vi "HandleObservationSync.vi"(8 "error in (no error)":errorcluster, 11 "S4GUI in":refnum<class "S4GUI.lvclass">) -> (0 "error out":errorcluster, 3 "S4GUI out":refnum<class "S4GUI.lvclass">)   [LabVIEW 2018, in "S4GUI.lvclass"] (continued)
                }
                frame True {
                  n489 = Concatenate Strings("CHANNEL ERROR " ("string"), ": Not idle. S4GUI:HandleObservationSync.vi state 252." ("Error Msg")) -> (w1188:string)
                }
              }
              n490 = Bundle By Name(cluster=w1171, "Obs_state"=w1169, "Error Msg"=w1162) -> (w1170:refnum<class "S4GUI.lvclass">)
            }
            frame 1 {
              n491 = Build Array(w1198, w1197, w1196, w1195) -> (w1200:bool[])
              n492 = Boolean Array To Number(Boolean array=w1200) -> (number=w1199:u32)
              n493 = Number To Decimal String(number=w1199) -> (decimal integer string=w1193:string)  [unwired: 1 in]
              n494 = Concatenate Strings("CHANNEL ERROR < " ("string"), w1193, ">: Initialization failed. S4GUI:HandleObservationSync.vi state 252." ("Error Msg")) -> (w1192:string)
              n495 = Bundle By Name(cluster=w1203, "Obs_state"=u32 1, "Error Msg"=w1192) -> (w1202:refnum<class "S4GUI.lvclass">)
            }
            frame 2 {
              n496 = Build Array(w1213, w1212, w1211, w1210) -> (w1209:bool[])
              n497 = Boolean Array To Number(Boolean array=w1209) -> (number=w1205:u32)
              n498 = Number To Decimal String(number=w1205) -> (decimal integer string=w1204:string)  [unwired: 1 in]
              n499 = Concatenate Strings("CHANNEL ERROR < " ("string"), w1204, ">:  Invalid Exposition Time. S4GUI:HandleObservationSync.vi state 252." ("Error Msg")) -> (w1207:string)
              n500 = Bundle By Name(cluster=w1216, "Obs_state"=u32 1, "Error Msg"=w1207) -> (w1215:refnum<class "S4GUI.lvclass">)
            }
            frame 3 {
              n501 = Bundle By Name(cluster=w1220, "Obs_state"=u32 1, "Error Msg"="ERROR: Invalid configuration in the channels. S4GUI:HandleObservationSync.vi state 252.") -> (w1219:refnum<class "S4GUI.lvclass">)
            }
          }
        }
        frame 253 {
          # "Sem SyncBox, \ntrigger mode = 0 (internal)\nCom SyncBox\ntrigger mode = 6 (ext. start)"
          n502 = call-dynamic "Read Sync Box.lvclass.vi"("error in (no error)"=w1332, "SPARC4_AC in"=w1331) -> ("error out"=w1334:errorcluster, "Sync Box.lvclass"=w1335:refnum<class "Sync Box.lvclass">, "SPARC4_AC out"=w1330:refnum<class "S4GUI.lvclass">)  [unwired: 7 in]
          n503 = call "Read connection.vi"("error in (no error)"=w1334, "Server in"=w1335) -> ("error out"=w1333:errorcluster, "connection"=w1295:bool)  [unwired: 7 in, 1 out]
          n504 = case shown="True" w1295 {
            tunnel: [u8 6 ("TRIGGER_MODE") u8 0 ("TRIGGER_MODE")] -> w1312
            frame True {
            }
            frame False {
            }
          }
          n505 = call-dynamic "Read AcquisitionA.vi"("error in (no error)"=w1333, "S4ACS_GUI in"=w1330) -> ("error out"=w1317:errorcluster, "Acquisition.lvclass"=w1318:refnum<class "Acquisition.lvclass">, "S4ACS_GUI out"=w1316:refnum<class "S4GUI.lvclass">)  [unwired: 7 in]
          n506 = call-dynamic "Read Channel.vi"("error in (no error)"=w1317, "Acquisition in"=w1318) -> ("error out"=w1300:errorcluster, "Channel.lvclass"=w1299:refnum<class "Channel.lvclass">, "Acquisition out"=w1327:refnum<class "Acquisition.lvclass">)  [unwired: 7 in]
          n507 = call-dynamic "Read Interface.vi"("error in (no error)"=w1300, "Channel in"=w1299) -> ("error out"=w1298:errorcluster, "Interface.lvclass"=w1304:refnum<class "Interface.lvclass">, "Channel out"=w1303:refnum<class "Channel.lvclass">)  [unwired: 7 in]
          n508 = call-dynamic "Get CCD_Config.vi"("error in (no error)"=w1298, "Interface in"=w1304) -> ("error out"=w1311:errorcluster, "output cluster"=w1313:T1, "Interface out"=w1310:refnum<class "Interface.lvclass">)  [unwired: 7 in]
          n509 = Bundle By Name(cluster=w1313, "TRIGGER_MODE"=w1312) -> (w1309:T1)
          n510 = call-dynamic "Set CCD_Config.vi"("error in (no error)"=w1311, "input cluster"=w1309, "Interface in"=w1310) -> ("error out"=w1307:errorcluster, "Interface out"=w1305:refnum<class "Interface.lvclass">)  [unwired: 7 in]
          n511 = Flatten To String(anything=w1309, error in (no error)=w1307) -> (data string=w1308:string, error out=w1306:errorcluster)  [unwired: 2 in, 1 out]
          n512 = call "Write flatted cluster.vi"("error in (no error)"=w1306, "flatted cluster"=w1308, "Interface in"=w1305) -> ("error out"=w1301:errorcluster, "Interface out"=w1302:refnum<class "Interface.lvclass">)  [unwired: 7 in]
          n513 = Increment(x=w1338) -> (x+1=w1337:u32)
          n514 = call-dynamic "Write Interface.vi"("error in (no error)"=w1301, "Interface.lvclass"=w1302, "Channel in"=w1303) -> ("error out"=w1297:errorcluster, "Channel out"=w1296:refnum<class "Channel.lvclass">)  [unwired: 7 in]
          n515 = call-dynamic "Read State Machine.vi"("error in (no error)"=w1297, "Device in"=w1296) -> ("error out"=w1324:errorcluster, "State Machine.lvclass"=w1326:refnum<class "State Machine.lvclass">, "Device out"=w1322:refnum<class "Channel.lvclass">)  [unwired: 7 in]
          n516 = call "Next State.vi"("error in (no error)"=w1324, "New_State"=60, "State Machine in"=w1326) -> ("error out"=w1319:errorcluster, "State Machine out"=w1320:refnum<class "State Machine.lvclass">)  [unwired: 7 in]
          n517 = call-dynamic "Write State Machine.vi"("error in (no error)"=w1319, "State Machine.lvclass"=w1320, "Device in"=w1322) -> ("error out"=w1321:errorcluster, "Device out"=w1323:refnum<class "Channel.lvclass">)  [unwired: 7 in]
          n518 = call-dynamic "Write Channel.vi"("error in (no error)"=w1321, "Channel.lvclass"=w1323, "Acquisition in"=w1327) -> ("error out"=w1314:errorcluster, "Acquisition out"=w1315:refnum<class "Acquisition.lvclass">)  [unwired: 7 in]
          n519 = call-dynamic "Write AcquisitionA.vi"("error in (no error)"=w1314, "Acquisition.lvclass"=w1315, "S4ACS_GUI in"=w1316) -> ("error out"=w1329:errorcluster, "S4ACS_GUI out"=w1328:refnum<class "S4GUI.lvclass">)  [unwired: 7 in]
          n520 = Bundle By Name(cluster=w1328, "Obs_state"=w1337) -> (w1336:refnum<class "S4GUI.lvclass">)
        }
        frame 254 {
          # "Espera terminar a execução do comando atual \nantes de ir ao proximo passo da Observação."
          n521 = call-dynamic "Read AcquisitionA.vi"("error in (no error)"=w1358, "S4ACS_GUI in"=w1359) -> ("error out"=w1364:errorcluster, "Acquisition.lvclass"=w1365:refnum<class "Acquisition.lvclass">, "S4ACS_GUI out"=w1361:refnum<class "S4GUI.lvclass">)  [unwired: 7 in]
          n522 = call-dynamic "Read Channel.vi"("error in (no error)"=w1364, "Acquisition in"=w1365) -> ("error out"=w1356:errorcluster, "Channel.lvclass"=w1355:refnum<class "Channel.lvclass">, "Acquisition out"=w1363:refnum<class "Acquisition.lvclass">)  [unwired: 7 in]
          n523 = call-dynamic "Read State Machine.vi"("error in (no error)"=w1356, "Device in"=w1355) -> ("error out"=w1347:errorcluster, "State Machine.lvclass"=w1349:refnum<class "State Machine.lvclass">, "Device out"=w1353:refnum<class "Channel.lvclass">)  [unwired: 7 in]
          n524 = call-dynamic "Read State.vi"("error in (no error)"=w1347, "State Machine in"=w1349) -> ("error out"=w1346:errorcluster, "State"=w1343:i32, "State Machine out"=w1348:refnum<class "State Machine.lvclass">)  [unwired: 7 in]
          n525 = Equal To 0?(x=w1343) -> (x = 0?=w1345:bool)
          n526 = call-dynamic "Write State Machine.vi"("error in (no error)"=w1346, "State Machine.lvclass"=w1348, "Device in"=w1353) -> ("error out"=w1352:errorcluster, "Device out"=w1354:refnum<class "Channel.lvclass">)  [unwired: 7 in]
          n527 = call-dynamic "Write Channel.vi"("error in (no error)"=w1352, "Channel.lvclass"=w1354, "Acquisition in"=w1363) -> ("error out"=w1360:errorcluster, "Acquisition out"=w1362:refnum<class "Acquisition.lvclass">)  [unwired: 7 in]
          n528 = disable-structure shown="Enabled" {
            disable-tunnel: [u32 299 ("t") w1367] -> w1342
            disable-tunnel: w1341 -> [_ w1368]
            frame Disabled {
            }
            frame Enabled {
              n529 = Increment(x=w1368) -> (x+1=w1367:u32)
            }
          }
          n530 = Select(t=w1342, s=w1345, f=w1341) -> (s? t:f=w1344:u32)
          n531 = call-dynamic "Write AcquisitionA.vi"("error in (no error)"=w1360, "Acquisition.lvclass"=w1362, "S4ACS_GUI in"=w1361) -> ("error out"=w1357:errorcluster, "S4ACS_GUI out"=w1351:refnum<class "S4GUI.lvclass">)  [unwired: 7 in]
          n532 = Bundle By Name(cluster=w1351, "Obs_state"=w1344) -> (w1350:refnum<class "S4GUI.lvclass">)
        }
        frame 255 {
          n533 = call "Read AcquisitionB.vi"("error in (no error)"=w1379, "S4ACS_GUI in"=w1380) -> ("error out"=w1372:errorcluster, "Acquisition.lvclass"=w1373:refnum<class "Acquisition.lvclass">, "S4ACS_GUI out"=w1382:refnum<class "S4GUI.lvclass">)  [unwired: 7 in]
          n534 = call "Read connection.vi"("error in (no error)"=w1372, "Server in"=w1373) -> ("error out"=w1371:errorcluster, "connection"=w1369:bool, "Server out"=w1370:refnum<class "Acquisition.lvclass">)  [unwired: 7 in]
          n535 = case shown="False" w1369 {
            tunnel: w1370 -> [w1390 w1410]
            tunnel: w1371 -> [w1389 w1409]
            tunnel: [w1390 w1407] -> w1383
            tunnel: [w1389 w1406] -> w1381
            tunnel: w1376 -> [w1388 w1399]
            tunnel: [w1384 w1398] -> w1375
            frame False {
              n536 = Increment(x=w1388) -> (x+1=w1387:u32)
              n537 = Increment(x=w1387) -> (x+1=w1386:u32)
              n538 = Increment(x=w1386) -> (x+1=w1385:u32)
              n539 = Increment(x=w1385) -> (x+1=w1384:u32)
            }
            frame True {
              # "configura o canal,\nmas não dispara\na exposicao."
              n540 = call-dynamic "Read Channel.vi"("error in (no error)"=w1409, "Acquisition in"=w1410) -> ("error out"=w1395:errorcluster, "Channel.lvclass"=w1397:refnum<class "Channel.lvclass">, "Acquisition out"=w1408:refnum<class "Acquisition.lvclass">)  [unwired: 7 in]
              n541 = call-dynamic "Write expose.vi"("error in (no error)"=w1395, "expose"=FALSE, "Channel in"=w1397) -> ("error out"=w1394:errorcluster, "Channel out"=w1396:refnum<class "Channel.lvclass">)  [unwired: 7 in]
              n542 = call-dynamic "Read State Machine.vi"("error in (no error)"=w1394, "Device in"=w1396) -> ("error out"=w1403:errorcluster, "State Machine.lvclass"=w1405:refnum<class "State Machine.lvclass">, "Device out"=w1401:refnum<class "Channel.lvclass">)  [unwired: 7 in]
              n543 = call "Next State.vi"("error in (no error)"=w1403, "New_State"=1, "State Machine in"=w1405) -> ("error out"=w1391:errorcluster, "State Machine out"=w1392:refnum<class "State Machine.lvclass">)  [unwired: 7 in]
              n544 = Increment(x=w1399) -> (x+1=w1398:u32)
              n545 = call-dynamic "Write State Machine.vi"("error in (no error)"=w1391, "State Machine.lvclass"=w1392, "Device in"=w1401) -> ("error out"=w1400:errorcluster, "Device out"=w1402:refnum<class "Channel.lvclass">)  [unwired: 7 in]
              n546 = call-dynamic "Write Channel.vi"("error in (no error)"=w1400, "Channel.lvclass"=w1402, "Acquisition in"=w1408) -> ("error out"=w1406:errorcluster, "Acquisition out"=w1407:refnum<class "Acquisition.lvclass">)  [unwired: 7 in]
            }
          }
          n547 = call "Write AcquisitionB.vi"("error in (no error)"=w1381, "Acquisition.lvclass"=w1383, "S4ACS_GUI in"=w1382) -> ("error out"=w1378:errorcluster, "S4ACS_GUI out"=w1377:refnum<class "S4GUI.lvclass">)  [unwired: 7 in]
          n548 = Bundle By Name(cluster=w1377, "Obs_state"=w1375) -> (w1374:refnum<class "S4GUI.lvclass">)
        }
        frame 256 {
          # "Espera terminar a execução do comando atual \nantes de ir ao proximo passo da Observação."
          n549 = call "Read AcquisitionB.vi"("error in (no error)"=w1428, "S4ACS_GUI in"=w1429) -> ("error out"=w1434:errorcluster, "Acquisition.lvclass"=w1435:refnum<class "Acquisition.lvclass">, "S4ACS_GUI out"=w1431:refnum<class "S4GUI.lvclass">)  [unwired: 7 in]
          n550 = call-dynamic "Read Channel.vi"("error in (no error)"=w1434, "Acquisition in"=w1435) -> ("error out"=w1426:errorcluster, "Channel.lvclass"=w1425:refnum<class "Channel.lvclass">, "Acquisition out"=w1433:refnum<class "Acquisition.lvclass">)  [unwired: 7 in]
          n551 = call-dynamic "Read State Machine.vi"("error in (no error)"=w1426, "Device in"=w1425) -> ("error out"=w1417:errorcluster, "State Machine.lvclass"=w1419:refnum<class "State Machine.lvclass">, "Device out"=w1423:refnum<class "Channel.lvclass">)  [unwired: 7 in]
          n552 = call-dynamic "Read State.vi"("error in (no error)"=w1417, "State Machine in"=w1419) -> ("error out"=w1416:errorcluster, "State"=w1413:i32, "State Machine out"=w1418:refnum<class "State Machine.lvclass">)  [unwired: 7 in]
          n553 = call-dynamic "Write State Machine.vi"("error in (no error)"=w1416, "State Machine.lvclass"=w1418, "Device in"=w1423) -> ("error out"=w1422:errorcluster, "Device out"=w1424:refnum<class "Channel.lvclass">)  [unwired: 7 in]
          n554 = call-dynamic "Write Channel.vi"("error in (no error)"=w1422, "Channel.lvclass"=w1424, "Acquisition in"=w1433) -> ("error out"=w1430:errorcluster, "Acquisition out"=w1432:refnum<class "Acquisition.lvclass">)  [unwired: 7 in]
          n555 = Equal To 0?(x=w1413) -> (x = 0?=w1415:bool)
          n556 = disable-structure shown="Enabled" {
            disable-tunnel: [u32 299 ("t") w1437] -> w1411
            disable-tunnel: w1412 -> [_ w1440]
            frame Disabled {
            }
            frame Enabled {
              n557 = Increment(x=w1440) -> (x+1=w1439:u32)
              n558 = Increment(x=w1439) -> (x+1=w1438:u32)
              n559 = Increment(x=w1438) -> (x+1=w1437:u32)
            }
          }
          n560 = Select(t=w1411, s=w1415, f=w1412) -> (s? t:f=w1414:u32)
          n561 = call "Write AcquisitionB.vi"("error in (no error)"=w1430, "Acquisition.lvclass"=w1432, "S4ACS_GUI in"=w1431) -> ("error out"=w1427:errorcluster, "S4ACS_GUI out"=w1421:refnum<class "S4GUI.lvclass">)  [unwired: 7 in]
          n562 = Bundle By Name(cluster=w1421, "Obs_state"=w1414) -> (w1420:refnum<class "S4GUI.lvclass">)
        }
        frame 257 {
          # "Sem SyncBox, \ntrigger mode = 0 (internal)\nCom SyncBox\ntrigger mode = 6 (ext. start)"
          n563 = call-dynamic "Read Sync Box.lvclass.vi"("error in (no error)"=w1478, "SPARC4_AC in"=w1477) -> ("error out"=w1480:errorcluster, "Sync Box.lvclass"=w1481:refnum<class "Sync Box.lvclass">, "SPARC4_AC out"=w1476:refnum<class "S4GUI.lvclass">)  [unwired: 7 in]
          n564 = call "Read connection.vi"("error in (no error)"=w1480, "Server in"=w1481) -> ("error out"=w1479:errorcluster, "connection"=w1442:bool)  [unwired: 7 in, 1 out]
          n565 = case shown="False" w1442 {
            tunnel: [u8 6 ("TRIGGER_MODE") u8 0 ("TRIGGER_MODE")] -> w1441
            frame True {
            }
            frame False {
            }
          }
          n566 = call "Read AcquisitionB.vi"("error in (no error)"=w1479, "S4ACS_GUI in"=w1476) -> ("error out"=w1463:errorcluster, "Acquisition.lvclass"=w1464:refnum<class "Acquisition.lvclass">, "S4ACS_GUI out"=w1462:refnum<class "S4GUI.lvclass">)  [unwired: 7 in]
          n567 = call-dynamic "Read Channel.vi"("error in (no error)"=w1463, "Acquisition in"=w1464) -> ("error out"=w1447:errorcluster, "Channel.lvclass"=w1446:refnum<class "Channel.lvclass">, "Acquisition out"=w1473:refnum<class "Acquisition.lvclass">)  [unwired: 7 in]
          n568 = call-dynamic "Read Interface.vi"("error in (no error)"=w1447, "Channel in"=w1446) -> ("error out"=w1445:errorcluster, "Interface.lvclass"=w1451:refnum<class "Interface.lvclass">, "Channel out"=w1450:refnum<class "Channel.lvclass">)  [unwired: 7 in]
          n569 = call-dynamic "Get CCD_Config.vi"("error in (no error)"=w1445, "Interface in"=w1451) -> ("error out"=w1458:errorcluster, "output cluster"=w1459:T1, "Interface out"=w1457:refnum<class "Interface.lvclass">)  [unwired: 7 in]
          n570 = Bundle By Name(cluster=w1459, "TRIGGER_MODE"=w1441) -> (w1456:T1)
          n571 = call-dynamic "Set CCD_Config.vi"("error in (no error)"=w1458, "input cluster"=w1456, "Interface in"=w1457) -> ("error out"=w1454:errorcluster, "Interface out"=w1452:refnum<class "Interface.lvclass">)  [unwired: 7 in]
          n572 = Flatten To String(anything=w1456, error in (no error)=w1454) -> (data string=w1455:string, error out=w1453:errorcluster)  [unwired: 2 in, 1 out]
          n573 = call "Write flatted cluster.vi"("error in (no error)"=w1453, "flatted cluster"=w1455, "Interface in"=w1452) -> ("error out"=w1448:errorcluster, "Interface out"=w1449:refnum<class "Interface.lvclass">)  [unwired: 7 in]
          n574 = Increment(x=w1484) -> (x+1=w1483:u32)
          n575 = call-dynamic "Write Interface.vi"("error in (no error)"=w1448, "Interface.lvclass"=w1449, "Channel in"=w1450) -> ("error out"=w1444:errorcluster, "Channel out"=w1443:refnum<class "Channel.lvclass">)  [unwired: 7 in]
          n576 = call-dynamic "Read State Machine.vi"("error in (no error)"=w1444, "Device in"=w1443) -> ("error out"=w1470:errorcluster, "State Machine.lvclass"=w1472:refnum<class "State Machine.lvclass">, "Device out"=w1468:refnum<class "Channel.lvclass">)  [unwired: 7 in]
          n577 = call "Next State.vi"("error in (no error)"=w1470, "New_State"=60, "State Machine in"=w1472) -> ("error out"=w1465:errorcluster, "State Machine out"=w1466:refnum<class "State Machine.lvclass">)  [unwired: 7 in]
          n578 = call-dynamic "Write State Machine.vi"("error in (no error)"=w1465, "State Machine.lvclass"=w1466, "Device in"=w1468) -> ("error out"=w1467:errorcluster, "Device out"=w1469:refnum<class "Channel.lvclass">)  [unwired: 7 in]
          n579 = call-dynamic "Write Channel.vi"("error in (no error)"=w1467, "Channel.lvclass"=w1469, "Acquisition in"=w1473) -> ("error out"=w1460:errorcluster, "Acquisition out"=w1461:refnum<class "Acquisition.lvclass">)  [unwired: 7 in]
          n580 = call "Write AcquisitionB.vi"("error in (no error)"=w1460, "Acquisition.lvclass"=w1461, "S4ACS_GUI in"=w1462) -> ("error out"=w1475:errorcluster, "S4ACS_GUI out"=w1474:refnum<class "S4GUI.lvclass">)  [unwired: 7 in]
          n581 = Bundle By Name(cluster=w1474, "Obs_state"=w1483) -> (w1482:refnum<class "S4GUI.lvclass">)
        }
        frame 258 {
          # "Espera terminar a execução do comando atual \nantes de ir ao proximo passo da Observação."
          n582 = call "Read AcquisitionB.vi"("error in (no error)"=w1504, "S4ACS_GUI in"=w1505) -> ("error out"=w1510:errorcluster, "Acquisition.lvclass"=w1511:refnum<class "Acquisition.lvclass">, "S4ACS_GUI out"=w1507:refnum<class "S4GUI.lvclass">)  [unwired: 7 in]
          n583 = call-dynamic "Read Channel.vi"("error in (no error)"=w1510, "Acquisition in"=w1511) -> ("error out"=w1502:errorcluster, "Channel.lvclass"=w1501:refnum<class "Channel.lvclass">, "Acquisition out"=w1509:refnum<class "Acquisition.lvclass">)  [unwired: 7 in]
          n584 = call-dynamic "Read State Machine.vi"("error in (no error)"=w1502, "Device in"=w1501) -> ("error out"=w1493:errorcluster, "State Machine.lvclass"=w1495:refnum<class "State Machine.lvclass">, "Device out"=w1499:refnum<class "Channel.lvclass">)  [unwired: 7 in]
          n585 = call-dynamic "Read State.vi"("error in (no error)"=w1493, "State Machine in"=w1495) -> ("error out"=w1492:errorcluster, "State"=w1489:i32, "State Machine out"=w1494:refnum<class "State Machine.lvclass">)  [unwired: 7 in]
          n586 = call-dynamic "Write State Machine.vi"("error in (no error)"=w1492, "State Machine.lvclass"=w1494, "Device in"=w1499) -> ("error out"=w1498:errorcluster, "Device out"=w1500:refnum<class "Channel.lvclass">)  [unwired: 7 in]
          n587 = call-dynamic "Write Channel.vi"("error in (no error)"=w1498, "Channel.lvclass"=w1500, "Acquisition in"=w1509) -> ("error out"=w1506:errorcluster, "Acquisition out"=w1508:refnum<class "Acquisition.lvclass">)  [unwired: 7 in]
          n588 = Equal To 0?(x=w1489) -> (x = 0?=w1491:bool)
          n589 = Increment(x=w1488) -> (x+1=w1487:u32)
          n590 = Select(t=w1487, s=w1491, f=w1488) -> (s? t:f=w1490:u32)
          n591 = call "Write AcquisitionB.vi"("error in (no error)"=w1506, "Acquisition.lvclass"=w1508, "S4ACS_GUI in"=w1507) -> ("error out"=w1503:errorcluster, "S4ACS_GUI out"=w1497:refnum<class "S4GUI.lvclass">)  [unwired: 7 in]
          n592 = Bundle By Name(cluster=w1497, "Obs_state"=w1490) -> (w1496:refnum<class "S4GUI.lvclass">)
        }
        frame 259 {
          n593 = call-dynamic "Read AcquisitionC.vi"("error in (no error)"=w1522, "S4ACS_GUI in"=w1523) -> ("error out"=w1514:errorcluster, "Acquisition.lvclass"=w1516:refnum<class "Acquisition.lvclass">, "S4ACS_GUI out"=w1525:refnum<class "S4GUI.lvclass">)  [unwired: 7 in]
          n594 = call "Read connection.vi"("error in (no error)"=w1514, "Server in"=w1516) -> ("error out"=w1513:errorcluster, "connection"=w1512:bool, "Server out"=w1515:refnum<class "Acquisition.lvclass">)  [unwired: 7 in]
          n595 = case shown="True" w1512 {
            tunnel: w1515 -> [w1532 w1553]
            tunnel: w1513 -> [w1533 w1552]
            tunnel: [w1532 w1550] -> w1526
            tunnel: [w1533 w1549] -> w1524
            tunnel: w1519 -> [w1531 w1542]
            tunnel: [w1527 w1541] -> w1518
            frame False {
              n596 = Increment(x=w1531) -> (x+1=w1530:u32)
              n597 = Increment(x=w1530) -> (x+1=w1529:u32)
              n598 = Increment(x=w1529) -> (x+1=w1528:u32)
              n599 = Increment(x=w1528) -> (x+1=w1527:u32)
            }
            frame True {
              # "configura o canal,\nmas não dispara\na exposicao."
              n600 = call-dynamic "Read Channel.vi"("error in (no error)"=w1552, "Acquisition in"=w1553) -> ("error out"=w1538:errorcluster, "Channel.lvclass"=w1540:refnum<class "Channel.lvclass">, "Acquisition out"=w1551:refnum<class "Acquisition.lvclass">)  [unwired: 7 in]
              n601 = call-dynamic "Write expose.vi"("error in (no error)"=w1538, "expose"=FALSE, "Channel in"=w1540) -> ("error out"=w1537:errorcluster, "Channel out"=w1539:refnum<class "Channel.lvclass">)  [unwired: 7 in]
              n602 = call-dynamic "Read State Machine.vi"("error in (no error)"=w1537, "Device in"=w1539) -> ("error out"=w1546:errorcluster, "State Machine.lvclass"=w1548:refnum<class "State Machine.lvclass">, "Device out"=w1544:refnum<class "Channel.lvclass">)  [unwired: 7 in]
              n603 = call "Next State.vi"("error in (no error)"=w1546, "New_State"=1, "State Machine in"=w1548) -> ("error out"=w1534:errorcluster, "State Machine out"=w1535:refnum<class "State Machine.lvclass">)  [unwired: 7 in]
              n604 = Increment(x=w1542) -> (x+1=w1541:u32)
              n605 = call-dynamic "Write State Machine.vi"("error in (no error)"=w1534, "State Machine.lvclass"=w1535, "Device in"=w1544) -> ("error out"=w1543:errorcluster, "Device out"=w1545:refnum<class "Channel.lvclass">)  [unwired: 7 in]
              n606 = call-dynamic "Write Channel.vi"("error in (no error)"=w1543, "Channel.lvclass"=w1545, "Acquisition in"=w1551) -> ("error out"=w1549:errorcluster, "Acquisition out"=w1550:refnum<class "Acquisition.lvclass">)  [unwired: 7 in]
            }
          }
          n607 = call-dynamic "Write AcquisitionC.vi"("error in (no error)"=w1524, "Acquisition.lvclass"=w1526, "S4ACS_GUI in"=w1525) -> ("error out"=w1521:errorcluster, "S4ACS_GUI out"=w1520:refnum<class "S4GUI.lvclass">)  [unwired: 7 in]
          n608 = Bundle By Name(cluster=w1520, "Obs_state"=w1518) -> (w1517:refnum<class "S4GUI.lvclass">)
        }
        frame 260 {
          # "Espera terminar a execução do comando atual \nantes de ir ao proximo passo da Observação."
          n609 = call-dynamic "Read AcquisitionC.vi"("error in (no error)"=w1571, "S4ACS_GUI in"=w1572) -> ("error out"=w1577:errorcluster, "Acquisition.lvclass"=w1578:refnum<class "Acquisition.lvclass">, "S4ACS_GUI out"=w1574:refnum<class "S4GUI.lvclass">)  [unwired: 7 in]
          n610 = call-dynamic "Read Channel.vi"("error in (no error)"=w1577, "Acquisition in"=w1578) -> ("error out"=w1569:errorcluster, "Channel.lvclass"=w1568:refnum<class "Channel.lvclass">, "Acquisition out"=w1576:refnum<class "Acquisition.lvclass">)  [unwired: 7 in]
          n611 = call-dynamic "Read State Machine.vi"("error in (no error)"=w1569, "Device in"=w1568) -> ("error out"=w1560:errorcluster, "State Machine.lvclass"=w1562:refnum<class "State Machine.lvclass">, "Device out"=w1566:refnum<class "Channel.lvclass">)  [unwired: 7 in]
          n612 = call-dynamic "Read State.vi"("error in (no error)"=w1560, "State Machine in"=w1562) -> ("error out"=w1559:errorcluster, "State"=w1556:i32, "State Machine out"=w1561:refnum<class "State Machine.lvclass">)  [unwired: 7 in]
          n613 = Equal To 0?(x=w1556) -> (x = 0?=w1558:bool)
          n614 = call-dynamic "Write State Machine.vi"("error in (no error)"=w1559, "State Machine.lvclass"=w1561, "Device in"=w1566) -> ("error out"=w1565:errorcluster, "Device out"=w1567:refnum<class "Channel.lvclass">)  [unwired: 7 in]
          n615 = call-dynamic "Write Channel.vi"("error in (no error)"=w1565, "Channel.lvclass"=w1567, "Acquisition in"=w1576) -> ("error out"=w1573:errorcluster, "Acquisition out"=w1575:refnum<class "Acquisition.lvclass">)  [unwired: 7 in]
          n616 = disable-structure shown="Enabled" {
            disable-tunnel: [u32 299 ("t") w1580] -> w1554
            disable-tunnel: w1555 -> [_ w1583]
            frame Disabled {
            }
            frame Enabled {
              n617 = Increment(x=w1583) -> (x+1=w1582:u32)
              n618 = Increment(x=w1582) -> (x+1=w1581:u32)
              n619 = Increment(x=w1581) -> (x+1=w1580:u32)
            }
          }
          n620 = Select(t=w1554, s=w1558, f=w1555) -> (s? t:f=w1557:u32)
          n621 = call-dynamic "Write AcquisitionC.vi"("error in (no error)"=w1573, "Acquisition.lvclass"=w1575, "S4ACS_GUI in"=w1574) -> ("error out"=w1570:errorcluster, "S4ACS_GUI out"=w1564:refnum<class "S4GUI.lvclass">)  [unwired: 7 in]
          n622 = Bundle By Name(cluster=w1564, "Obs_state"=w1557) -> (w1563:refnum<class "S4GUI.lvclass">)
        }
        frame 261 {
          # "Sem SyncBox, \ntrigger mode = 0 (internal)\nCom SyncBox\ntrigger mode = 6 (ext. start)"
          n623 = call-dynamic "Read Sync Box.lvclass.vi"("error in (no error)"=w1621, "SPARC4_AC in"=w1620) -> ("error out"=w1623:errorcluster, "Sync Box.lvclass"=w1624:refnum<class "Sync Box.lvclass">, "SPARC4_AC out"=w1619:refnum<class "S4GUI.lvclass">)  [unwired: 7 in]
          n624 = call "Read connection.vi"("error in (no error)"=w1623, "Server in"=w1624) -> ("error out"=w1622:errorcluster, "connection"=w1585:bool)  [unwired: 7 in, 1 out]
          n625 = case shown="False" w1585 {
            tunnel: [u8 6 ("TRIGGER_MODE") u8 0 ("TRIGGER_MODE")] -> w1584
            frame True {
            }
            frame False {
            }
          }
          n626 = call-dynamic "Read AcquisitionC.vi"("error in (no error)"=w1622, "S4ACS_GUI in"=w1619) -> ("error out"=w1606:errorcluster, "Acquisition.lvclass"=w1607:refnum<class "Acquisition.lvclass">, "S4ACS_GUI out"=w1605:refnum<class "S4GUI.lvclass">)  [unwired: 7 in]
          n627 = call-dynamic "Read Channel.vi"("error in (no error)"=w1606, "Acquisition in"=w1607) -> ("error out"=w1590:errorcluster, "Channel.lvclass"=w1589:refnum<class "Channel.lvclass">, "Acquisition out"=w1616:refnum<class "Acquisition.lvclass">)  [unwired: 7 in]
          n628 = call-dynamic "Read Interface.vi"("error in (no error)"=w1590, "Channel in"=w1589) -> ("error out"=w1588:errorcluster, "Interface.lvclass"=w1594:refnum<class "Interface.lvclass">, "Channel out"=w1593:refnum<class "Channel.lvclass">)  [unwired: 7 in]
          n629 = call-dynamic "Get CCD_Config.vi"("error in (no error)"=w1588, "Interface in"=w1594) -> ("error out"=w1601:errorcluster, "output cluster"=w1602:T1, "Interface out"=w1600:refnum<class "Interface.lvclass">)  [unwired: 7 in]
          n630 = Bundle By Name(cluster=w1602, "TRIGGER_MODE"=w1584) -> (w1599:T1)
          n631 = call-dynamic "Set CCD_Config.vi"("error in (no error)"=w1601, "input cluster"=w1599, "Interface in"=w1600) -> ("error out"=w1597:errorcluster, "Interface out"=w1595:refnum<class "Interface.lvclass">)  [unwired: 7 in]
          n632 = Flatten To String(anything=w1599, error in (no error)=w1597) -> (data string=w1598:string, error out=w1596:errorcluster)  [unwired: 2 in, 1 out]
          n633 = call "Write flatted cluster.vi"("error in (no error)"=w1596, "flatted cluster"=w1598, "Interface in"=w1595) -> ("error out"=w1591:errorcluster, "Interface out"=w1592:refnum<class "Interface.lvclass">)  [unwired: 7 in]
          n634 = Increment(x=w1627) -> (x+1=w1626:u32)
          n635 = call-dynamic "Write Interface.vi"("error in (no error)"=w1591, "Interface.lvclass"=w1592, "Channel in"=w1593) -> ("error out"=w1587:errorcluster, "Channel out"=w1586:refnum<class "Channel.lvclass">)  [unwired: 7 in]
          n636 = call-dynamic "Read State Machine.vi"("error in (no error)"=w1587, "Device in"=w1586) -> ("error out"=w1613:errorcluster, "State Machine.lvclass"=w1615:refnum<class "State Machine.lvclass">, "Device out"=w1611:refnum<class "Channel.lvclass">)  [unwired: 7 in]
          n637 = call "Next State.vi"("error in (no error)"=w1613, "New_State"=60, "State Machine in"=w1615) -> ("error out"=w1608:errorcluster, "State Machine out"=w1609:refnum<class "State Machine.lvclass">)  [unwired: 7 in]
          n638 = call-dynamic "Write State Machine.vi"("error in (no error)"=w1608, "State Machine.lvclass"=w1609, "Device in"=w1611) -> ("error out"=w1610:errorcluster, "Device out"=w1612:refnum<class "Channel.lvclass">)  [unwired: 7 in]
          n639 = call-dynamic "Write Channel.vi"("error in (no error)"=w1610, "Channel.lvclass"=w1612, "Acquisition in"=w1616) -> ("error out"=w1603:errorcluster, "Acquisition out"=w1604:refnum<class "Acquisition.lvclass">)  [unwired: 7 in]
          n640 = call-dynamic "Write AcquisitionC.vi"("error in (no error)"=w1603, "Acquisition.lvclass"=w1604, "S4ACS_GUI in"=w1605) -> ("error out"=w1618:errorcluster, "S4ACS_GUI out"=w1617:refnum<class "S4GUI.lvclass">)  [unwired: 7 in]
          n641 = Bundle By Name(cluster=w1617, "Obs_state"=w1626) -> (w1625:refnum<class "S4GUI.lvclass">)
        }
        frame 262 {
          # "Espera terminar a execução do comando atual \nantes de ir ao proximo passo da Observação."
          n642 = call-dynamic "Read AcquisitionC.vi"("error in (no error)"=w1647, "S4ACS_GUI in"=w1648) -> ("error out"=w1653:errorcluster, "Acquisition.lvclass"=w1654:refnum<class "Acquisition.lvclass">, "S4ACS_GUI out"=w1650:refnum<class "S4GUI.lvclass">)  [unwired: 7 in]
          n643 = call-dynamic "Read Channel.vi"("error in (no error)"=w1653, "Acquisition in"=w1654) -> ("error out"=w1645:errorcluster, "Channel.lvclass"=w1644:refnum<class "Channel.lvclass">, "Acquisition out"=w1652:refnum<class "Acquisition.lvclass">)  [unwired: 7 in]
          n644 = call-dynamic "Read State Machine.vi"("error in (no error)"=w1645, "Device in"=w1644) -> ("error out"=w1636:errorcluster, "State Machine.lvclass"=w1638:refnum<class "State Machine.lvclass">, "Device out"=w1642:refnum<class "Channel.lvclass">)  [unwired: 7 in]
          n645 = call-dynamic "Read State.vi"("error in (no error)"=w1636, "State Machine in"=w1638) -> ("error out"=w1635:errorcluster, "State"=w1632:i32, "State Machine out"=w1637:refnum<class "State Machine.lvclass">)  [unwired: 7 in]
          n646 = Equal To 0?(x=w1632) -> (x = 0?=w1634:bool)
          n647 = call-dynamic "Write State Machine.vi"("error in (no error)"=w1635, "State Machine.lvclass"=w1637, "Device in"=w1642) -> ("error out"=w1641:errorcluster, "Device out"=w1643:refnum<class "Channel.lvclass">)  [unwired: 7 in]
          n648 = call-dynamic "Write Channel.vi"("error in (no error)"=w1641, "Channel.lvclass"=w1643, "Acquisition in"=w1652) -> ("error out"=w1649:errorcluster, "Acquisition out"=w1651:refnum<class "Acquisition.lvclass">)  [unwired: 7 in]
          n649 = Increment(x=w1631) -> (x+1=w1630:u32)
          n650 = Select(t=w1630, s=w1634, f=w1631) -> (s? t:f=w1633:u32)
          n651 = call-dynamic "Write AcquisitionC.vi"("error in (no error)"=w1649, "Acquisition.lvclass"=w1651, "S4ACS_GUI in"=w1650) -> ("error out"=w1646:errorcluster, "S4ACS_GUI out"=w1640:refnum<class "S4GUI.lvclass">)  [unwired: 7 in]
          n652 = Bundle By Name(cluster=w1640, "Obs_state"=w1633) -> (w1639:refnum<class "S4GUI.lvclass">)
        }
        frame 263 {
          # "Dispara o comando para o dispositivo corrente."
          n653 = call-dynamic "Read AcquisitionD.vi"("error in (no error)"=w1665, "S4ACS_GUI in"=w1666) -> ("error out"=w1658:errorcluster, "Acquisition.lvclass"=w1659:refnum<class "Acquisition.lvclass">, "S4ACS_GUI out"=w1668:refnum<class "S4GUI.lvclass">)  [unwired: 7 in]
          n654 = call "Read connection.vi"("error in (no error)"=w1658, "Server in"=w1659) -> ("error out"=w1656:errorcluster, "connection"=w1655:bool, "Server out"=w1657:refnum<class "Acquisition.lvclass">)  [unwired: 7 in]
          n655 = case shown="True" w1655 {
            tunnel: w1657 -> [w1672 w1692]
            tunnel: w1656 -> [w1671 w1691]
            tunnel: [w1672 w1689] -> w1669
            tunnel: [w1671 w1688] -> w1667
            tunnel: w1662 -> [_ w1681]
            tunnel: [u32 299 w1680] -> w1661
            frame False {
            }
            frame True {
              # "configura o canal,\nmas não dispara\na exposicao."
              n656 = call-dynamic "Read Channel.vi"("error in (no error)"=w1691, "Acquisition in"=w1692) -> ("error out"=w1677:errorcluster, "Channel.lvclass"=w1679:refnum<class "Channel.lvclass">, "Acquisition out"=w1690:refnum<class "Acquisition.lvclass">)  [unwired: 7 in]
              n657 = call-dynamic "Write expose.vi"("error in (no error)"=w1677, "expose"=FALSE, "Channel in"=w1679) -> ("error out"=w1676:errorcluster, "Channel out"=w1678:refnum<class "Channel.lvclass">)  [unwired: 7 in]
              n658 = call-dynamic "Read State Machine.vi"("error in (no error)"=w1676, "Device in"=w1678) -> ("error out"=w1685:errorcluster, "State Machine.lvclass"=w1687:refnum<class "State Machine.lvclass">, "Device out"=w1683:refnum<class "Channel.lvclass">)  [unwired: 7 in]
              n659 = call "Next State.vi"("error in (no error)"=w1685, "New_State"=1, "State Machine in"=w1687) -> ("error out"=w1673:errorcluster, "State Machine out"=w1674:refnum<class "State Machine.lvclass">)  [unwired: 7 in]
              n660 = Increment(x=w1681) -> (x+1=w1680:u32)
              n661 = call-dynamic "Write State Machine.vi"("error in (no error)"=w1673, "State Machine.lvclass"=w1674, "Device in"=w1683) -> ("error out"=w1682:errorcluster, "Device out"=w1684:refnum<class "Channel.lvclass">)  [unwired: 7 in]
              n662 = call-dynamic "Write Channel.vi"("error in (no error)"=w1682, "Channel.lvclass"=w1684, "Acquisition in"=w1690) -> ("error out"=w1688:errorcluster, "Acquisition out"=w1689:refnum<class "Acquisition.lvclass">)  [unwired: 7 in]
            }
          }
          n663 = call-dynamic "Write AcquisitionD.vi"("error in (no error)"=w1667, "Acquisition.lvclass"=w1669, "S4ACS_GUI in"=w1668) -> ("error out"=w1664:errorcluster, "S4ACS_GUI out"=w1663:refnum<class "S4GUI.lvclass">)  [unwired: 7 in]
          n664 = Bundle By Name(cluster=w1663, "Obs_state"=w1661) -> (w1660:refnum<class "S4GUI.lvclass">)
        }
        frame 264 {
          # "Espera terminar a execução do comando atual \nantes de ir ao proximo passo da Observação."
          n665 = call-dynamic "Read AcquisitionD.vi"("error in (no error)"=w1710, "S4ACS_GUI in"=w1711) -> ("error out"=w1716:errorcluster, "Acquisition.lvclass"=w1717:refnum<class "Acquisition.lvclass">, "S4ACS_GUI out"=w1713:refnum<class "S4GUI.lvclass">)  [unwired: 7 in]
          n666 = call-dynamic "Read Channel.vi"("error in (no error)"=w1716, "Acquisition in"=w1717) -> ("error out"=w1708:errorcluster, "Channel.lvclass"=w1707:refnum<class "Channel.lvclass">, "Acquisition out"=w1715:refnum<class "Acquisition.lvclass">)  [unwired: 7 in]
          n667 = call-dynamic "Read State Machine.vi"("error in (no error)"=w1708, "Device in"=w1707) -> ("error out"=w1699:errorcluster, "State Machine.lvclass"=w1701:refnum<class "State Machine.lvclass">, "Device out"=w1705:refnum<class "Channel.lvclass">)  [unwired: 7 in]
          n668 = call-dynamic "Read State.vi"("error in (no error)"=w1699, "State Machine in"=w1701) -> ("error out"=w1698:errorcluster, "State"=w1695:i32, "State Machine out"=w1700:refnum<class "State Machine.lvclass">)  [unwired: 7 in]
          n669 = Equal To 0?(x=w1695) -> (x = 0?=w1697:bool)
          n670 = call-dynamic "Write State Machine.vi"("error in (no error)"=w1698, "State Machine.lvclass"=w1700, "Device in"=w1705) -> ("error out"=w1704:errorcluster, "Device out"=w1706:refnum<class "Channel.lvclass">)  [unwired: 7 in]
          n671 = call-dynamic "Write Channel.vi"("error in (no error)"=w1704, "Channel.lvclass"=w1706, "Acquisition in"=w1715) -> ("error out"=w1712:errorcluster, "Acquisition out"=w1714:refnum<class "Acquisition.lvclass">)  [unwired: 7 in]
          n672 = disable-structure shown="Enabled" {
            disable-tunnel: w1694 -> [w1719 _]
            disable-tunnel: [w1718 u32 299] -> w1693
            frame Disabled {
              n673 = Increment(x=w1719) -> (x+1=w1718:u32)
            }
            frame Enabled {
            }
          }
          n674 = Select(t=w1693, s=w1697, f=w1694) -> (s? t:f=w1696:u32)
          n675 = call-dynamic "Write AcquisitionD.vi"("error in (no error)"=w1712, "Acquisition.lvclass"=w1714, "S4ACS_GUI in"=w1713) -> ("error out"=w1709:errorcluster, "S4ACS_GUI out"=w1703:refnum<class "S4GUI.lvclass">)  [unwired: 7 in]
          n676 = Bundle By Name(cluster=w1703, "Obs_state"=w1696) -> (w1702:refnum<class "S4GUI.lvclass">)
        }
        frame 265 {
          # "Sem SyncBox, \ntrigger mode = 0 (internal)\nCom SyncBox\ntrigger mode = 6 (ext. start)"
          n677 = call-dynamic "Read Sync Box.lvclass.vi"("error in (no error)"=w1758, "SPARC4_AC in"=w1757) -> ("error out"=w1760:errorcluster, "Sync Box.lvclass"=w1761:refnum<class "Sync Box.lvclass">, "SPARC4_AC out"=w1756:refnum<class "S4GUI.lvclass">)  [unwired: 7 in]
          n678 = call "Read connection.vi"("error in (no error)"=w1760, "Server in"=w1761) -> ("error out"=w1759:errorcluster, "connection"=w1722:bool)  [unwired: 7 in, 1 out]
          n679 = case shown="False" w1722 {
            tunnel: [u8 6 ("TRIGGER_MODE") u8 0 ("TRIGGER_MODE")] -> w1721
            frame True {
            }
            frame False {
            }
          }
          n680 = call-dynamic "Read AcquisitionD.vi"("error in (no error)"=w1759, "S4ACS_GUI in"=w1756) -> ("error out"=w1743:errorcluster, "Acquisition.lvclass"=w1744:refnum<class "Acquisition.lvclass">, "S4ACS_GUI out"=w1742:refnum<class "S4GUI.lvclass">)  [unwired: 7 in]
          n681 = call-dynamic "Read Channel.vi"("error in (no error)"=w1743, "Acquisition in"=w1744) -> ("error out"=w1727:errorcluster, "Channel.lvclass"=w1726:refnum<class "Channel.lvclass">, "Acquisition out"=w1753:refnum<class "Acquisition.lvclass">)  [unwired: 7 in]
          n682 = call-dynamic "Read Interface.vi"("error in (no error)"=w1727, "Channel in"=w1726) -> ("error out"=w1725:errorcluster, "Interface.lvclass"=w1731:refnum<class "Interface.lvclass">, "Channel out"=w1730:refnum<class "Channel.lvclass">)  [unwired: 7 in]
          n683 = call-dynamic "Get CCD_Config.vi"("error in (no error)"=w1725, "Interface in"=w1731) -> ("error out"=w1738:errorcluster, "output cluster"=w1739:T1, "Interface out"=w1737:refnum<class "Interface.lvclass">)  [unwired: 7 in]
          n684 = Bundle By Name(cluster=w1739, "TRIGGER_MODE"=w1721) -> (w1736:T1)
          n685 = call-dynamic "Set CCD_Config.vi"("error in (no error)"=w1738, "input cluster"=w1736, "Interface in"=w1737) -> ("error out"=w1734:errorcluster, "Interface out"=w1732:refnum<class "Interface.lvclass">)  [unwired: 7 in]
          n686 = Flatten To String(anything=w1736, error in (no error)=w1734) -> (data string=w1735:string, error out=w1733:errorcluster)  [unwired: 2 in, 1 out]
          n687 = call "Write flatted cluster.vi"("error in (no error)"=w1733, "flatted cluster"=w1735, "Interface in"=w1732) -> ("error out"=w1728:errorcluster, "Interface out"=w1729:refnum<class "Interface.lvclass">)  [unwired: 7 in]
          n688 = call-dynamic "Write Interface.vi"("error in (no error)"=w1728, "Interface.lvclass"=w1729, "Channel in"=w1730) -> ("error out"=w1724:errorcluster, "Channel out"=w1723:refnum<class "Channel.lvclass">)  [unwired: 7 in]
          n689 = call-dynamic "Read State Machine.vi"("error in (no error)"=w1724, "Device in"=w1723) -> ("error out"=w1750:errorcluster, "State Machine.lvclass"=w1752:refnum<class "State Machine.lvclass">, "Device out"=w1748:refnum<class "Channel.lvclass">)  [unwired: 7 in]
          n690 = Increment(x=w1764) -> (x+1=w1763:u32)
          n691 = call "Next State.vi"("error in (no error)"=w1750, "New_State"=60, "State Machine in"=w1752) -> ("error out"=w1745:errorcluster, "State Machine out"=w1746:refnum<class "State Machine.lvclass">)  [unwired: 7 in]
          n692 = call-dynamic "Write State Machine.vi"("error in (no error)"=w1745, "State Machine.lvclass"=w1746, "Device in"=w1748) -> ("error out"=w1747:errorcluster, "Device out"=w1749:refnum<class "Channel.lvclass">)  [unwired: 7 in]
          n693 = call-dynamic "Write Channel.vi"("error in (no error)"=w1747, "Channel.lvclass"=w1749, "Acquisition in"=w1753) -> ("error out"=w1740:errorcluster, "Acquisition out"=w1741:refnum<class "Acquisition.lvclass">)  [unwired: 7 in]
          n694 = call-dynamic "Write AcquisitionD.vi"("error in (no error)"=w1740, "Acquisition.lvclass"=w1741, "S4ACS_GUI in"=w1742) -> ("error out"=w1755:errorcluster, "S4ACS_GUI out"=w1754:refnum<class "S4GUI.lvclass">)  [unwired: 7 in]
          n695 = Bundle By Name(cluster=w1754, "Obs_state"=w1763) -> (w1762:refnum<class "S4GUI.lvclass">)
        }
        frame 266 {
          # "Espera terminar a execução do comando atual \nantes de ir ao proximo passo da Observação."
          n696 = call-dynamic "Read AcquisitionD.vi"("error in (no error)"=w1784, "S4ACS_GUI in"=w1785) -> ("error out"=w1790:errorcluster, "Acquisition.lvclass"=w1791:refnum<class "Acquisition.lvclass">, "S4ACS_GUI out"=w1787:refnum<class "S4GUI.lvclass">)  [unwired: 7 in]
          n697 = call-dynamic "Read Channel.vi"("error in (no error)"=w1790, "Acquisition in"=w1791) -> ("error out"=w1782:errorcluster, "Channel.lvclass"=w1781:refnum<class "Channel.lvclass">, "Acquisition out"=w1789:refnum<class "Acquisition.lvclass">)  [unwired: 7 in]
          n698 = call-dynamic "Read State Machine.vi"("error in (no error)"=w1782, "Device in"=w1781) -> ("error out"=w1773:errorcluster, "State Machine.lvclass"=w1775:refnum<class "State Machine.lvclass">, "Device out"=w1779:refnum<class "Channel.lvclass">)  [unwired: 7 in]
          n699 = call-dynamic "Read State.vi"("error in (no error)"=w1773, "State Machine in"=w1775) -> ("error out"=w1772:errorcluster, "State"=w1769:i32, "State Machine out"=w1774:refnum<class "State Machine.lvclass">)  [unwired: 7 in]
          n700 = Equal To 0?(x=w1769) -> (x = 0?=w1771:bool)
          n701 = call-dynamic "Write State Machine.vi"("error in (no error)"=w1772, "State Machine.lvclass"=w1774, "Device in"=w1779) -> ("error out"=w1778:errorcluster, "Device out"=w1780:refnum<class "Channel.lvclass">)  [unwired: 7 in]
          n702 = call-dynamic "Write Channel.vi"("error in (no error)"=w1778, "Channel.lvclass"=w1780, "Acquisition in"=w1789) -> ("error out"=w1786:errorcluster, "Acquisition out"=w1788:refnum<class "Acquisition.lvclass">)  [unwired: 7 in]
          n703 = Select(t=u32 299, s=w1771, f=w1768) -> (s? t:f=w1770:u32)
          n704 = call-dynamic "Write AcquisitionD.vi"("error in (no error)"=w1786, "Acquisition.lvclass"=w1788, "S4ACS_GUI in"=w1787) -> ("error out"=w1783:errorcluster, "S4ACS_GUI out"=w1777:refnum<class "S4GUI.lvclass">)  [unwired: 7 in]
          n705 = Bundle By Name(cluster=w1777, "Obs_state"=w1770) -> (w1776:refnum<class "S4GUI.lvclass">)
        }
        frame 271 {
          # "Prepara os canais de aquisição para sequencia de foco...."
          n706 = flat-sequence {
            tunnel: w1818 -> [w1923]
            tunnel: [w1923] -> w1817
            frame #0 {
              n707 = Tick Count (ms)() -> (millisecond timer value=→"time5":u32)
            }
          }
          n708 = call-dynamic "Read AcquisitionA.vi"("error in (no error)"=w1817, "S4ACS_GUI in"=w1839) -> ("error out"=w1837:errorcluster, "Acquisition.lvclass"=w1838:refnum<class "Acquisition.lvclass">, "S4ACS_GUI out"=w1841:refnum<class "S4GUI.lvclass">)  [unwired: 7 in]
          n709 = call "Read connection.vi"("error in (no error)"=w1837, "Server in"=w1838) -> ("error out"=w1836:errorcluster, "connection"=w1816:bool, "Server out"=w1835:refnum<class "Acquisition.lvclass">)  [unwired: 7 in]
          n710 = case shown="True" w1816 {
            tunnel: [w1904 w1922] -> w1842
            tunnel: [w1903 w1921] -> w1840
            tunnel: w1836 -> [w1903 w1920]
            tunnel: w1835 -> [w1904 w1919]
            frame False {
            }
            frame True {
              # "configura o canal,\nmas não dispara\na exposicao."
              n711 = call-dynamic "Read Channel.vi"("error in (no error)"=w1920, "Acquisition in"=w1919) -> ("error out"=w1909:errorcluster, "Channel.lvclass"=w1911:refnum<class "Channel.lvclass">, "Acquisition out"=w1918:refnum<class "Acquisition.lvclass">)  [unwired: 7 in]
              n712 = call-dynamic "Write expose.vi"("error in (no error)"=w1909, "expose"=FALSE, "Channel in"=w1911) -> ("error out"=w1908:errorcluster, "Channel out"=w1910:refnum<class "Channel.lvclass">)  [unwired: 7 in]
              n713 = call-dynamic "Read State Machine.vi"("error in (no error)"=w1908, "Device in"=w1910) -> ("error out"=w1915:errorcluster, "State Machine.lvclass"=w1917:refnum<class "State Machine.lvclass">, "Device out"=w1913:refnum<class "Channel.lvclass">)  [unwired: 7 in]
              n714 = call "Next State.vi"("error in (no error)"=w1915, "New_State"=1, "State Machine in"=w1917) -> ("error out"=w1905:errorcluster, "State Machine out"=w1906:refnum<class "State Machine.lvclass">)  [unwired: 7 in]
              n715 = call-dynamic "Write State Machine.vi"("error in (no error)"=w1905, "State Machine.lvclass"=w1906, "Device in"=w1913) -> ("error out"=w1912:errorcluster, "Device out"=w1914:refnum<class "Channel.lvclass">)  [unwired: 7 in]
              n716 = call-dynamic "Write Channel.vi"("error in (no error)"=w1912, "Channel.lvclass"=w1914, "Acquisition in"=w1918) -> ("error out"=w1921:errorcluster, "Acquisition out"=w1922:refnum<class "Acquisition.lvclass">)  [unwired: 7 in]
            }
          }
          n717 = Increment(x=w1834) -> (x+1=w1798:u32)
          n718 = call-dynamic "Write AcquisitionA.vi"("error in (no error)"=w1840, "Acquisition.lvclass"=w1842, "S4ACS_GUI in"=w1841) -> ("error out"=w1830:errorcluster, "S4ACS_GUI out"=w1829:refnum<class "S4GUI.lvclass">)  [unwired: 7 in]
          n719 = call "Read AcquisitionB.vi"("error in (no error)"=w1830, "S4ACS_GUI in"=w1829) -> ("error out"=w1831:errorcluster, "Acquisition.lvclass"=w1832:refnum<class "Acquisition.lvclass">, "S4ACS_GUI out"=w1833:refnum<class "S4GUI.lvclass">)  [unwired: 7 in]
          n720 = call "Read connection.vi"("error in (no error)"=w1831, "Server in"=w1832) -> ("error out"=w1814:errorcluster, "connection"=w1813:bool, "Server out"=w1815:refnum<class "Acquisition.lvclass">)  [unwired: 7 in]
          n721 = case shown="True" w1813 {
            tunnel: [w1884 w1902] -> w1812
            tunnel: [w1883 w1901] -> w1811
            tunnel: w1814 -> [w1883 w1900]
            tunnel: w1815 -> [w1884 w1899]
            frame False {
            }
            frame True {
              # "configura o canal,\nmas não dispara\na exposicao."
              n722 = call-dynamic "Read Channel.vi"("error in (no error)"=w1900, "Acquisition in"=w1899) -> ("error out"=w1889:errorcluster, "Channel.lvclass"=w1891:refnum<class "Channel.lvclass">, "Acquisition out"=w1898:refnum<class "Acquisition.lvclass">)  [unwired: 7 in]
              n723 = call-dynamic "Write expose.vi"("error in (no error)"=w1889, "expose"=FALSE, "Channel in"=w1891) -> ("error out"=w1888:errorcluster, "Channel out"=w1890:refnum<class "Channel.lvclass">)  [unwired: 7 in]
              n724 = call-dynamic "Read State Machine.vi"("error in (no error)"=w1888, "Device in"=w1890) -> ("error out"=w1895:errorcluster, "State Machine.lvclass"=w1897:refnum<class "State Machine.lvclass">, "Device out"=w1893:refnum<class "Channel.lvclass">)  [unwired: 7 in]
              n725 = call "Next State.vi"("error in (no error)"=w1895, "New_State"=1, "State Machine in"=w1897) -> ("error out"=w1885:errorcluster, "State Machine out"=w1886:refnum<class "State Machine.lvclass">)  [unwired: 7 in]
              n726 = call-dynamic "Write State Machine.vi"("error in (no error)"=w1885, "State Machine.lvclass"=w1886, "Device in"=w1893) -> ("error out"=w1892:errorcluster, "Device out"=w1894:refnum<class "Channel.lvclass">)  [unwired: 7 in]
              n727 = call-dynamic "Write Channel.vi"("error in (no error)"=w1892, "Channel.lvclass"=w1894, "Acquisition in"=w1898) -> ("error out"=w1901:errorcluster, "Acquisition out"=w1902:refnum<class "Acquisition.lvclass">)  [unwired: 7 in]
            }
          }
          n728 = call "Write AcquisitionB.vi"("error in (no error)"=w1811, "Acquisition.lvclass"=w1812, "S4ACS_GUI in"=w1833) -> ("error out"=w1822:errorcluster, "S4ACS_GUI out"=w1821:refnum<class "S4GUI.lvclass">)  [unwired: 7 in]
          n729 = call-dynamic "Read AcquisitionC.vi"("error in (no error)"=w1822, "S4ACS_GUI in"=w1821) -> ("error out"=w1826:errorcluster, "Acquisition.lvclass"=w1827:refnum<class "Acquisition.lvclass">, "S4ACS_GUI out"=w1828:refnum<class "S4GUI.lvclass">)  [unwired: 7 in]
          n730 = call "Read connection.vi"("error in (no error)"=w1826, "Server in"=w1827) -> ("error out"=w1808:errorcluster, "connection"=w1809:bool, "Server out"=w1810:refnum<class "Acquisition.lvclass">)  [unwired: 7 in]
          n731 = case shown="True" w1809 {
            tunnel: [w1864 w1882] -> w1807
            tunnel: [w1863 w1881] -> w1806
            tunnel: w1808 -> [w1863 w1880]
            tunnel: w1810 -> [w1864 w1879]
            frame False {
            }
            frame True {
              # "configura o canal,\nmas não dispara\na exposicao."
              n732 = call-dynamic "Read Channel.vi"("error in (no error)"=w1880, "Acquisition in"=w1879) -> ("error out"=w1869:errorcluster, "Channel.lvclass"=w1871:refnum<class "Channel.lvclass">, "Acquisition out"=w1878:refnum<class "Acquisition.lvclass">)  [unwired: 7 in]
              n733 = call-dynamic "Write expose.vi"("error in (no error)"=w1869, "expose"=FALSE, "Channel in"=w1871) -> ("error out"=w1868:errorcluster, "Channel out"=w1870:refnum<class "Channel.lvclass">)  [unwired: 7 in]
              n734 = call-dynamic "Read State Machine.vi"("error in (no error)"=w1868, "Device in"=w1870) -> ("error out"=w1875:errorcluster, "State Machine.lvclass"=w1877:refnum<class "State Machine.lvclass">, "Device out"=w1873:refnum<class "Channel.lvclass">)  [unwired: 7 in]
              n735 = call "Next State.vi"("error in (no error)"=w1875, "New_State"=1, "State Machine in"=w1877) -> ("error out"=w1865:errorcluster, "State Machine out"=w1866:refnum<class "State Machine.lvclass">)  [unwired: 7 in]
              n736 = call-dynamic "Write State Machine.vi"("error in (no error)"=w1865, "State Machine.lvclass"=w1866, "Device in"=w1873) -> ("error out"=w1872:errorcluster, "Device out"=w1874:refnum<class "Channel.lvclass">)  [unwired: 7 in]
              n737 = call-dynamic "Write Channel.vi"("error in (no error)"=w1872, "Channel.lvclass"=w1874, "Acquisition in"=w1878) -> ("error out"=w1881:errorcluster, "Acquisition out"=w1882:refnum<class "Acquisition.lvclass">)  [unwired: 7 in]
            }
          }
          n738 = call-dynamic "Write AcquisitionC.vi"("error in (no error)"=w1806, "Acquisition.lvclass"=w1807, "S4ACS_GUI in"=w1828) -> ("error out"=w1820:errorcluster, "S4ACS_GUI out"=w1819:refnum<class "S4GUI.lvclass">)  [unwired: 7 in]
          n739 = call-dynamic "Read AcquisitionD.vi"("error in (no error)"=w1820, "S4ACS_GUI in"=w1819) -> ("error out"=w1823:errorcluster, "Acquisition.lvclass"=w1824:refnum<class "Acquisition.lvclass">, "S4ACS_GUI out"=w1825:refnum<class "S4GUI.lvclass">)  [unwired: 7 in]
          n740 = call "Read connection.vi"("error in (no error)"=w1823, "Server in"=w1824) -> ("error out"=w1803:errorcluster, "connection"=w1805:bool, "Server out"=w1804:refnum<class "Acquisition.lvclass">)  [unwired: 7 in]
          n741 = case shown="True" w1805 {
            tunnel: [w1844 w1862] -> w1802
            tunnel: [w1843 w1861] -> w1801
            tunnel: w1803 -> [w1843 w1860]
            tunnel: w1804 -> [w1844 w1859]
            frame False {
            }
            frame True {
              # "configura o canal,\nmas não dispara\na exposicao."
              n742 = call-dynamic "Read Channel.vi"("error in (no error)"=w1860, "Acquisition in"=w1859) -> ("error out"=w1849:errorcluster, "Channel.lvclass"=w1851:refnum<class "Channel.lvclass">, "Acquisition out"=w1858:refnum<class "Acquisition.lvclass">)  [unwired: 7 in]
              n743 = call-dynamic "Write expose.vi"("error in (no error)"=w1849, "expose"=FALSE, "Channel in"=w1851) -> ("error out"=w1848:errorcluster, "Channel out"=w1850:refnum<class "Channel.lvclass">)  [unwired: 7 in]
              n744 = call-dynamic "Read State Machine.vi"("error in (no error)"=w1848, "Device in"=w1850) -> ("error out"=w1855:errorcluster, "State Machine.lvclass"=w1857:refnum<class "State Machine.lvclass">, "Device out"=w1853:refnum<class "Channel.lvclass">)  [unwired: 7 in]
              n745 = call "Next State.vi"("error in (no error)"=w1855, "New_State"=1, "State Machine in"=w1857) -> ("error out"=w1845:errorcluster, "State Machine out"=w1846:refnum<class "State Machine.lvclass">)  [unwired: 7 in]
              n746 = call-dynamic "Write State Machine.vi"("error in (no error)"=w1845, "State Machine.lvclass"=w1846, "Device in"=w1853) -> ("error out"=w1852:errorcluster, "Device out"=w1854:refnum<class "Channel.lvclass">)  [unwired: 7 in]
              n747 = call-dynamic "Write Channel.vi"("error in (no error)"=w1852, "Channel.lvclass"=w1854, "Acquisition in"=w1858) -> ("error out"=w1861:errorcluster, "Acquisition out"=w1862:refnum<class "Acquisition.lvclass">)  [unwired: 7 in]
            }
          }
          n748 = call-dynamic "Write AcquisitionD.vi"("error in (no error)"=w1801, "Acquisition.lvclass"=w1802, "S4ACS_GUI in"=w1825) -> ("error out"=w1793:errorcluster, "S4ACS_GUI out"=w1797:refnum<class "S4GUI.lvclass">)  [unwired: 7 in]
          n749 = Unbundle By Name(w1797) -> ("TelFocus.lvclass"=w1796:refnum<class "TelFocus.lvclass">)
          n750 = call-dynamic "Write focus #stepsdone.vi"("error in (no error)"=w1793, "focus #stepsdone"=u32 0, "TelFocus in"=w1796) -> ("error out"=w1792:errorcluster, "TelFocus out"=w1794:refnum<class "TelFocus.lvclass">)  [unwired: 7 in]
          n751 = Bundle By Name(cluster=w1797, "TelFocus.lvclass"=w1794, "Error Msg"="", "Obs_state"=w1798) -> (w1799:refnum<class "S4GUI.lvclass">)
        }
        frame 272 {
          w1933 = 38 ("x")
          w1942 = 28 ("x")
          # "Se algum canal foi pra 38: Texp inválido \npara a configuração do CCD."
          # "Se algum canal foi pra 28: ERRO na inicialização."
          # "Espera terminar a execução da preparação\ndos 4 canais antes de ir ao proximo passo \nda Observação."
          n752 = flat-sequence {
            tunnel: w1975 -> [w2080]
            tunnel: [w2080] -> w1974
            frame #0 {
              n753 = Tick Count (ms)() -> (millisecond timer value=→"time6":u32)
            }
          }
          n754 = call-dynamic "Read AcquisitionA.vi"("error in (no error)"=w1974, "S4ACS_GUI in"=w1985) -> ("error out"=w1972:errorcluster, "Acquisition.lvclass"=w1973:refnum<class "Acquisition.lvclass">, "S4ACS_GUI out"=w1987:refnum<class "S4GUI.lvclass">)  [unwired: 7 in]
          n755 = call "Read connection.vi"("error in (no error)"=w1972, "Server in"=w1973) -> ("error out"=w1970:errorcluster, "connection"=w1969:bool, "Server out"=w1971:refnum<class "Acquisition.lvclass">)  [unwired: 7 in]
          n756 = case shown="True" w1969 {
            tunnel: w1971 -> [w2063 w2079]
            tunnel: w1970 -> [w2062 w2078]
            tunnel: [w2063 w2076] -> w1988
            tunnel: [w2062 w2075] -> w1986
            tunnel: [0 ("State") w2065] -> w1932
            frame False {
            }
            frame True {
              n757 = call-dynamic "Read Channel.vi"("error in (no error)"=w2078, "Acquisition in"=w2079) -> ("error out"=w2074:errorcluster, "Channel.lvclass"=w2073:refnum<class "Channel.lvclass">, "Acquisition out"=w2077:refnum<class "Acquisition.lvclass">)  [unwired: 7 in]
              n758 = call-dynamic "Read State Machine.vi"("error in (no error)"=w2074, "Device in"=w2073) -> ("error out"=w2067:errorcluster, "State Machine.lvclass"=w2069:refnum<class "State Machine.lvclass">, "Device out"=w2071:refnum<class "Channel.lvclass">)  [unwired: 7 in]
              n759 = call-dynamic "Read State.vi"("error in (no error)"=w2067, "State Machine in"=w2069) -> ("error out"=w2066:errorcluster, "State"=w2065:i32, "State Machine out"=w2068:refnum<class "State Machine.lvclass">)  [unwired: 7 in]
              n760 = call-dynamic "Write State Machine.vi"("error in (no error)"=w2066, "State Machine.lvclass"=w2068, "Device in"=w2071) -> ("error out"=w2070:errorcluster, "Device out"=w2072:refnum<class "Channel.lvclass">)  [unwired: 7 in]
